vi "MakeExample.vi"(8 "error in (no error)":errorcluster, 9 "TriggerRefractoryPeriod (Frames)":i32, 10 "StimulusObject Parameters":variant, 11 "FullWormRailsTwoColors in":refnum<class "FullWormRailsTwoColors.lvclass">) -> (0 "error out":errorcluster, 3 "FullWormRailsTwoColors out":refnum<class "FullWormRailsTwoColors.lvclass">)   [LabVIEW 2019, in "FullWormRailsTwoColors.lvclass"]
uses:
  FullWormRailsTwoColors.lvclass
  FullWormRailsTwoColorsInputCluster.ctl
  FullWormRailsTwoColors.lvclass/FullWormRailsTwoColors.ctl
  ParametersGlobal.vi
  StimulusObject.lvclass
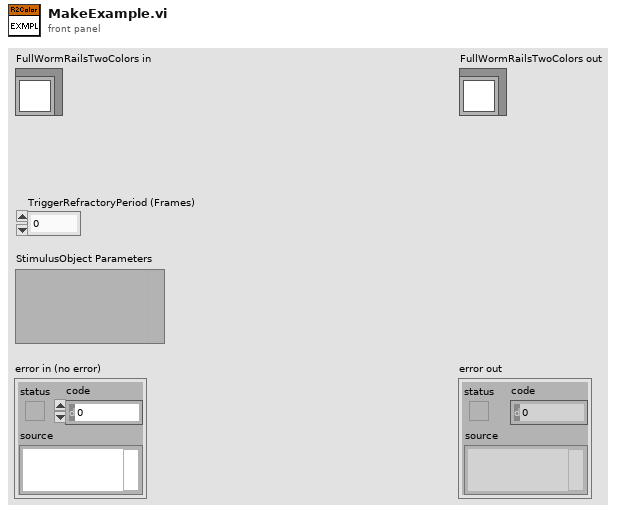
[diagram p1: front panel]
types:
  T1 = typedef "FullWormRailsTwoColors.lvclass/FullWormRailsTwoColorsInputCluster.ctl" = cluster{"Constant Intensity (uW/mm^2, negative is blue)":sgl, "dot radius (mm)":sgl, "BlueIntensity (uW/mm^2, negative is blue)":sgl[], "Durations (s)":sgl[], "Inter trigger interval (s)":dbl, "RedIntensity (uW/mm^2, positive is red)":sgl[]}
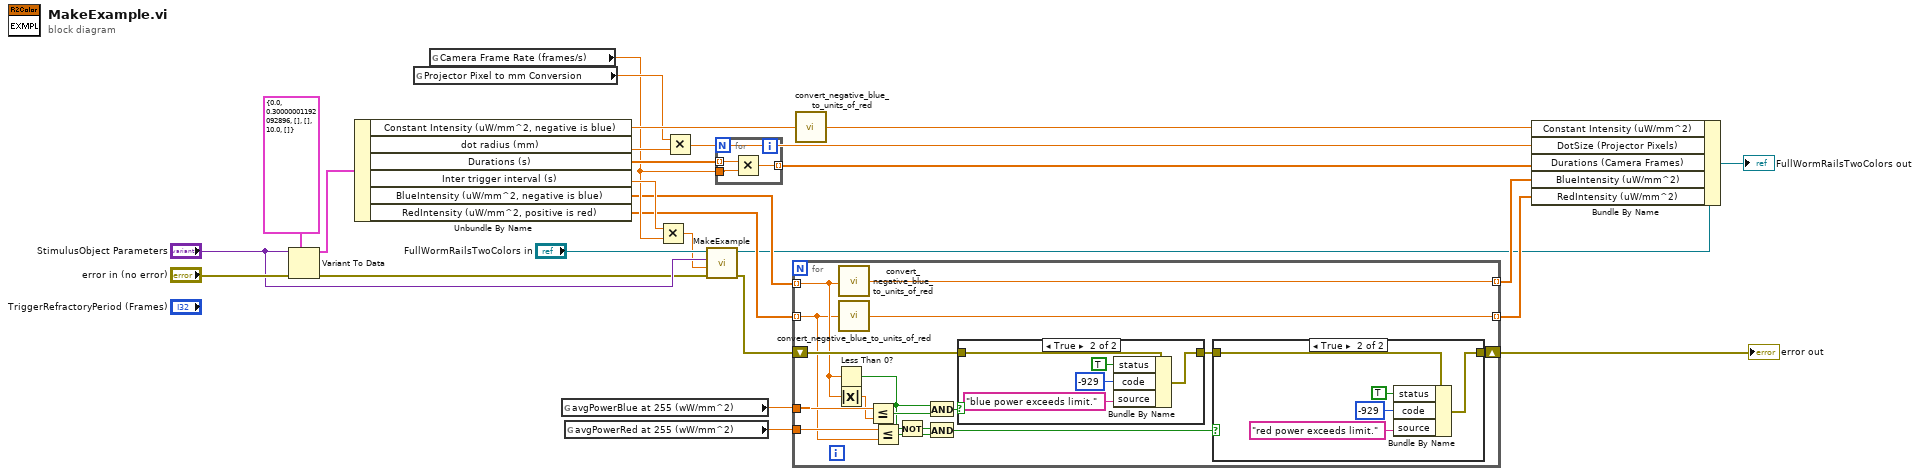
[diagram p0: block diagram]
diagram:
  n1 = Variant To Data(error in="error in (no error)", type=T1 {"Constant Intensity (uW/mm^2, negative is blue)"=0.0, "dot radius (mm)"=0.3, "BlueIntensity (uW/mm^2, negative is blue)"=[], "Durations (s)"=[], "Inter trigger interval (s)"=10.0, "RedIntensity (uW/mm^2, positive is red)"=[]} ("FullWormRailsTwoColorsInputCluster"), Variant="StimulusObject Parameters") -> (data=w26:T1, error out=w1:errorcluster)
  n2 = Unbundle By Name(w26) -> ("Constant Intensity (uW/mm^2, negative is blue)"=w24:sgl, "dot radius (mm)"=w22:sgl, "Durations (s)"=w19:sgl[], "Inter trigger interval (s)"=w25:dbl, "BlueIntensity (uW/mm^2, negative is blue)"=w14:sgl[], "RedIntensity (uW/mm^2, positive is red)"=w12:sgl[])
  n3 = global read "ParametersGlobal.vi" "Projector Pixel to mm Conversion"() -> (w21:sgl)
  n4 = global read "ParametersGlobal.vi" "Camera Frame Rate (frames/s)"() -> (w18:sgl)
  n5 = global read "ParametersGlobal.vi" "avgPowerBlue at 255 (wW/mm^2)"() -> (w16:sgl)
  n6 = global read "ParametersGlobal.vi" "avgPowerRed at 255 (wW/mm^2)"() -> (w15:sgl)
  n7 = Multiply(x=w25, y=w18) -> (x*y=w2:dbl)
  n8 = Multiply(x=w21, y=w22) -> (x*y=w20:sgl)
  n9 = call-parent "MakeExample.vi"("error in (no error)"=w1, "TriggerRefractoryPeriod (Frames)"=w2, "StimulusObject Parameters"="StimulusObject Parameters", "StimulusObject in"="FullWormRailsTwoColors in") -> ("error out"=w4:errorcluster, "StimulusObject out"=w5:refnum<class "FullWormRailsTwoColors.lvclass">)  [unwired: 6 in]
  n10 = for {
    tunnel: w19 -> [w29] mode=indexing
    tunnel: w18 -> [w28]
    tunnel: [w27] -> w17 mode=indexing
    n11 = Multiply(x=w29, y=w28) -> (x*y=w27:sgl)
  }
  n12 = for {
    tunnel: w14 -> [w32] mode=indexing
    shift-right: [w43] -> w7
    shift-left: w4 -> [w44]
    tunnel: w16 -> [w42]
    tunnel: w15 -> [w41]
    tunnel: [w40] -> w13 mode=indexing
    tunnel: w12 -> [w30] mode=indexing
    tunnel: [w31] -> w11 mode=indexing
    n13 = Less Than 0?(x=w32) -> (x < 0?=w33:bool)
    n14 = Absolute Value(x=w32) -> (abs(x)=w39:sgl)
    n15 = call "convert_negative_blue_to_units_of_red.vi"("Intensity in units of red (positive) and blue (negative)"=w32) -> ("Intensity in units of red (positive and negative)"=w40:sgl)
    n16 = call "convert_negative_blue_to_units_of_red.vi"("Intensity in units of red (positive) and blue (negative)"=w30) -> ("Intensity in units of red (positive and negative)"=w31:sgl)
    n17 = Less Or Equal?(x=w42, y=w39) -> (x <= y?=w38:bool)
    n18 = Less Or Equal?(x=w41, y=w30) -> (x <= y?=w35:bool)
    n19 = Not(x=w33) -> (.not. x?=w34:bool)
    n20 = And(x=w33, y=w38) -> (x .and. y?=w37:bool)
    n21 = And(x=w34, y=w35) -> (x .and. y?=w36:bool)
    n22 = case shown="True" w37 {
      tunnel: w44 -> [w52 w57]
      tunnel: [w52 w56] -> w45
      frame False {
      }
      frame True {
        n23 = Bundle By Name(cluster=w57, "status"=TRUE, "code"=-929, "source"="blue power exceeds limit.") -> (w56:errorcluster)
      }
    }
    n24 = case shown="True" w36 {
      tunnel: w45 -> [w46 w51]
      tunnel: [w46 w50] -> w43
      frame False {
      }
      frame True {
        n25 = Bundle By Name(cluster=w51, "status"=TRUE, "code"=-929, "source"="red power exceeds limit.") -> (w50:errorcluster)
      }
    }
  }
  "error out" <- w7
  n26 = call "convert_negative_blue_to_units_of_red.vi"("Intensity in units of red (positive) and blue (negative)"=w24) -> ("Intensity in units of red (positive and negative)"=w23:sgl)
  n27 = Bundle By Name(cluster=w5, "Constant Intensity (uW/mm^2)"=w23, "DotSize (Projector Pixels)"=w20, "Durations (Camera Frames)"=w17, "BlueIntensity (uW/mm^2)"=w13, "RedIntensity (uW/mm^2)"=w11) -> (→"FullWormRailsTwoColors out":refnum<class "FullWormRailsTwoColors.lvclass">)
